vi "读取零件名称.vi"(8 "error in (no error)":errorcluster caption="错误输入（无错误）", 11 "零件加工（抽象）输入":refnum<class "零件加工（抽象）.lvclass">) -> (0 "error out":errorcluster caption="错误输出", 2 "零件名称":string, 3 "零件加工（抽象）输出":refnum<class "零件加工（抽象）.lvclass">)   [LabVIEW 2013, in "零件加工（抽象）.lvclass"]
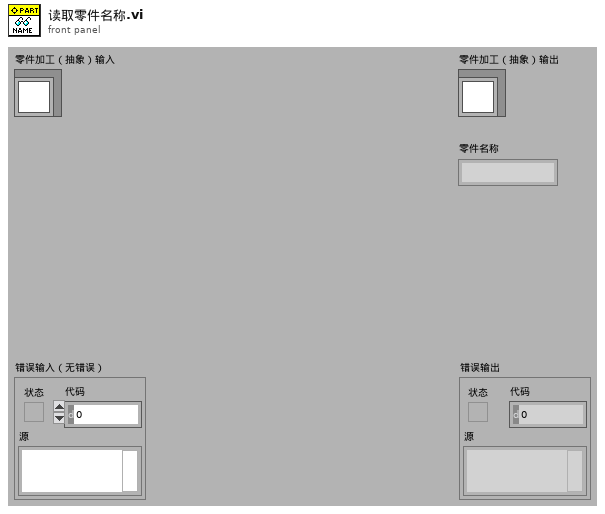
[diagram p1: front panel]
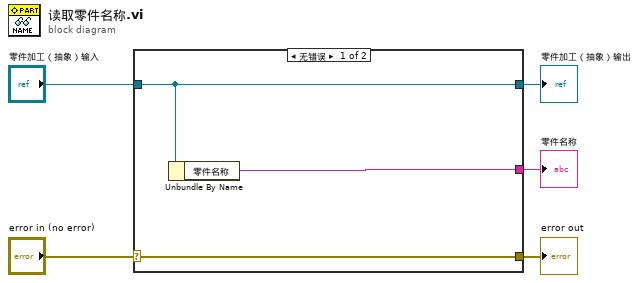
[diagram p0: block diagram]
diagram:
  n1 = case shown="无错误" "error in (no error)" {
    selector: "error in (no error)" -> [w8 w9]
    tunnel: [w8 w9] -> w4
    tunnel: [w7 w10] -> w2
    tunnel: "零件加工（抽象）输入" -> [w7 w10]
    tunnel: [w6 _] -> w1
    frame No Error {
      n2 = Unbundle By Name(w7) -> ("零件名称"=w6:string)
    }
    frame Error {
    }
  }
  "error out" <- w4
  "零件加工（抽象）输出" <- w2
  "零件名称" <- w1
